vi "start.vi"(8 "error in (no error)":errorcluster, 11 "QuadraturePositionDecoder in":refnum<class "QuadraturePositionDecoder.lvclass">) -> (0 "error out":errorcluster, 3 "QuadraturePositionDecoder out":refnum<class "QuadraturePositionDecoder.lvclass">)   [LabVIEW 2014, in "QuadraturePositionDecoder.lvclass"]
uses:
  QuadraturePositionDecoder.lvclass
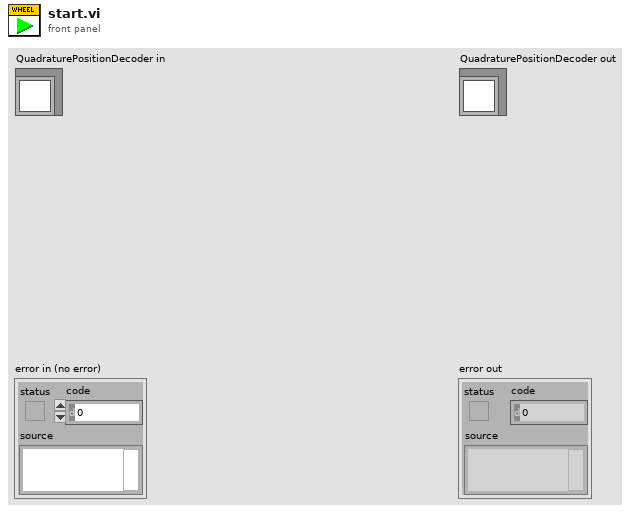
[diagram p1: front panel]
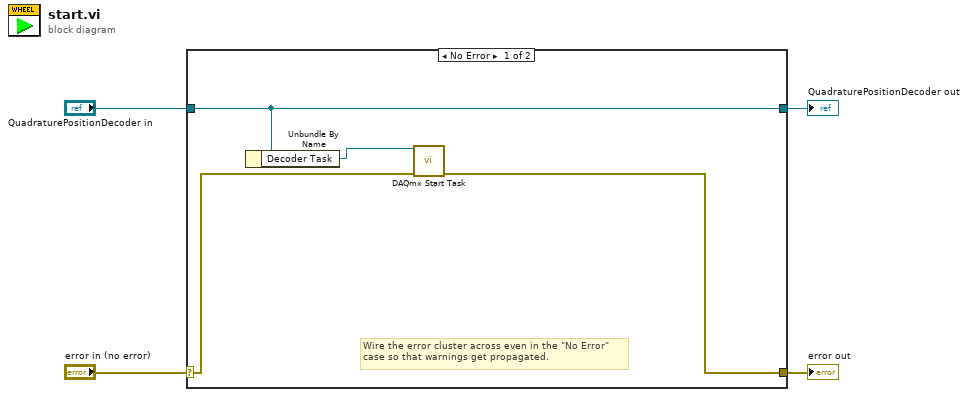
[diagram p0: block diagram]
diagram:
  n1 = case shown="No Error" "error in (no error)" {
    selector: "error in (no error)" -> [w6 w10]
    tunnel: [w5 w10] -> w3
    tunnel: [w8 w9] -> w1
    tunnel: "QuadraturePositionDecoder in" -> [w8 w9]
    frame No Error {
      # "Wire the error cluster across even in the \"No Error\"\ncase so that warnings get propagated."
      n2 = Unbundle By Name(w8) -> ("Decoder Task"=w7:refnum<k21>)
      n3 = call <vilib>:"DAQmx Start Task.vi"("task/channels in"=w7, "error in"=w6) -> ("error out"=w5:errorcluster)  [unwired: 12 in, 1 out]
    }
    frame Error {
    }
  }
  "error out" <- w3
  "QuadraturePositionDecoder out" <- w1
